vi "Task Start.vi"(8 "error in (no error)":errorcluster, 11 "ChartGuiTask in":refnum<class "ChartGuiTask.lvclass">) -> (0 "error out":errorcluster, 3 "ChartGuiTask out":refnum<class "ChartGuiTask.lvclass">)   [LabVIEW 2020, in "VolatusDemo.lvlib" / "ChartGuiTask.lvclass"]
uses:
  ChartGuiTask.lvclass
  ChartGuiTask.lvclass/ChartGuiTask.ctl
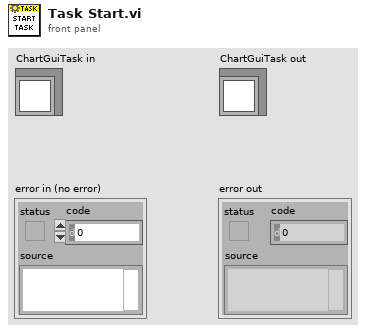
[diagram p1: front panel]
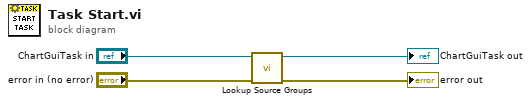
[diagram p0: block diagram]
diagram:
  n1 = call "Lookup Source Groups.vi"("error in (no error)"="error in (no error)", "ChartGuiTask in"="ChartGuiTask in") -> ("error out"=→"error out":errorcluster, "ChartGuiTask out"=→"ChartGuiTask out":refnum<class "ChartGuiTask.lvclass">)  [unwired: 8 in]
